vi "Test 5 Example Data 3.vi"(8 "error in (no error)":errorcluster, 11 "Test Case In":refnum<class "Tests Rev2.lvclass">) -> (0 "error out":errorcluster, 3 "Test Case Out":refnum<class "Tests Rev2.lvclass">)   [LabVIEW 2021, in "Tests Rev2.lvclass"]
uses:
  Tests Rev2.lvclass
  Tests Rev2.lvclass/Tests Rev2.ctl
  4993e8ee-a06a-463a-9684-69129f64d5ce.vi
  Proto/Group.lvclass
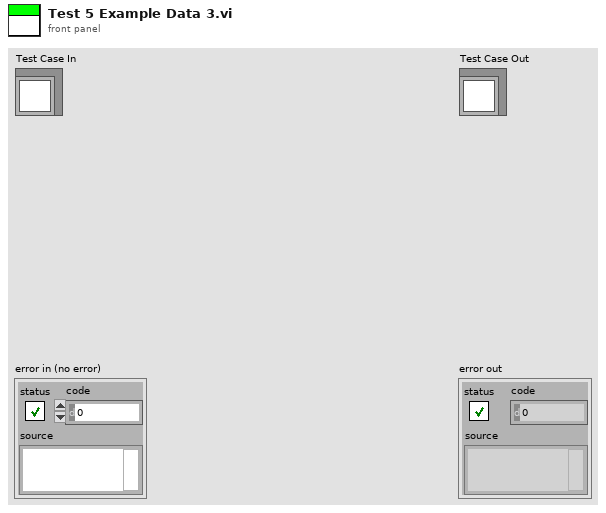
[diagram p1: front panel]
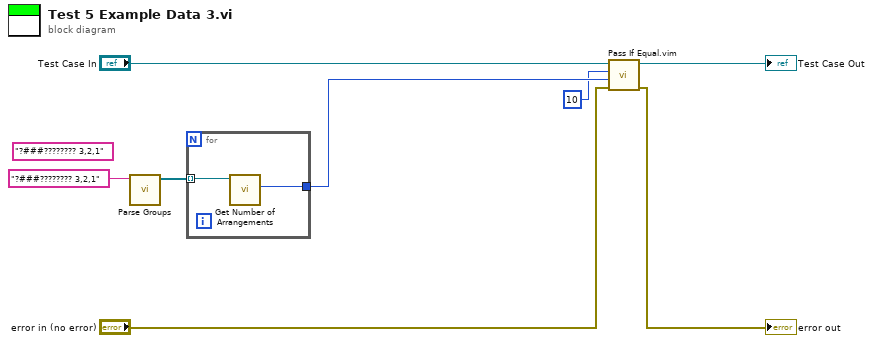
[diagram p0: block diagram]
diagram:
  (unwired) "?###???????? 3,2,1" ("Input")
  n1 = call "Parse Groups.vi"("Input"="?###???????? 3,2,1") -> ("Groups"=w2:refnum<class "Group.lvclass">[])  [unwired: 10 in]
  n2 = for {
    tunnel: [w10] -> w4
    tunnel: w2 -> [w9] mode=indexing
    n3 = call "Get Number of Arrangements.vi"("Proto in"=w9) -> ("Arrangements"=w10:u64)  [unwired: 8 in, 2 out]
  }
  n4 = call "Pass If Equal.vim"("error in (no error)"="error in (no error)", "Actual"=w4, "Expected"=u64 10 ("Arrangements"), "LUnit Test Case In"="Test Case In") -> ("error out"=→"error out":errorcluster, "LUnit Test Case Out"=→"Test Case Out":refnum<class "Tests Rev2.lvclass">)  [unwired: 6 in]
